vi "XML_GetAllAttributeValues.vi"(8 "Error In":errorcluster, 10 "Attribute Names to find[]":string[](array[string]), 11 "Node Refnum (In)":refnum<k20>) -> (0 "Error Out":errorcluster, 3 "Attribute Values[]":string[](array[string]))   [LabVIEW 2014]
uses:
  <resource>/objmgr/DOMUserDefRef.rc
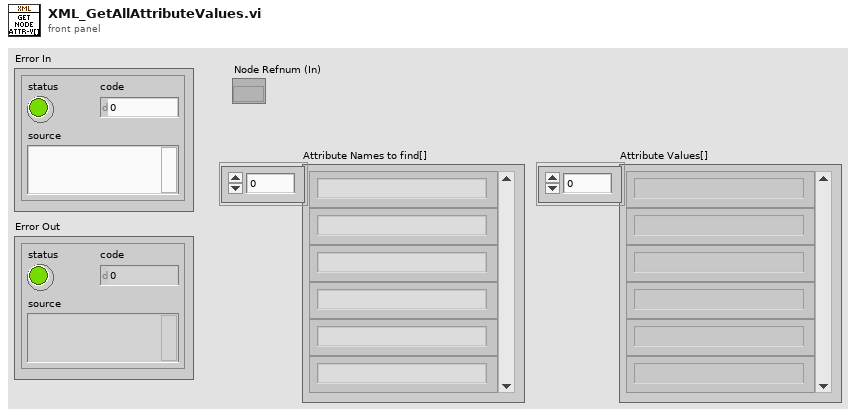
[diagram p1: front panel]
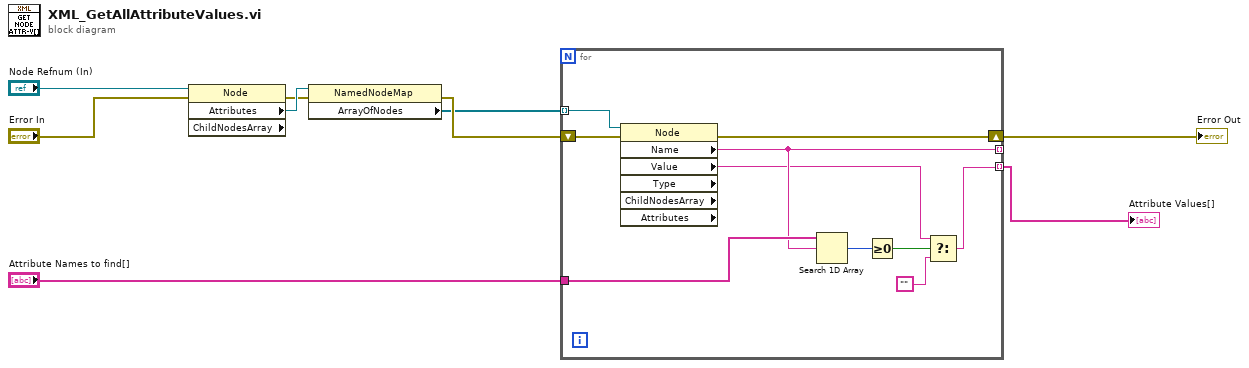
[diagram p0: block diagram]
diagram:
  n1 = property class="Node" props=["Attributes", "ChildNodesArray"](reference="Node Refnum (In)", error in="Error In") -> (error out=w3:errorcluster, "Attributes"=w9:refnum<k20>)  [unwired: 2 out]
  n2 = property class="NamedNodeMap"(reference=w9, error in=w3) -> (error out=w2:errorcluster, "ArrayOfNodes"=w1:refnum<k20>[])  [unwired: 1 out]
  n3 = for {
    tunnel: w1 -> [w10] mode=indexing
    tunnel: [w11] -> w7 mode=indexing
    tunnel: [w16] -> _ mode=indexing
    shift-right: [w18] -> w6
    shift-left: w2 -> [w19]
    tunnel: "Attribute Names to find[]" -> [w17]
    n4 = property class="Node" props=["Name", "Value", "Type", "ChildNodesArray", "Attributes"](reference=w10, error in=w19) -> (error out=w18:errorcluster, "Name"=w16:string, "Value"=w13:string)  [unwired: 4 out]
    n5 = Search 1D Array(1D array=w17, element=w16) -> (index of element=w15:i32)  [unwired: 1 in]
    n6 = Greater Or Equal To 0?(x=w15) -> (x >= 0?=w14:bool)
    n7 = Select(t=w13, s=w14, f="") -> (s? t:f=w11:string)
  }
  "Attribute Values[]" <- w7
  "Error Out" <- w6
